vi "READDB.vi"(8 "error in (no error)":errorcluster) -> (0 "error out":errorcluster, 1 "IDS":string[](array[string]), 2 "Datos":string[][](table) caption="Result Set (from first statement with results)", 3 "Max ID":i32)   [LabVIEW 2020, in "Settings.lvlib"]
uses:
  Settings.lvlib
  <vilib>/drjdpowell/SQLite Library/SQL Connection/Open (path).vi
  <vilib>/drjdpowell/SQLite Library/SQL Connection/Open (string).vi
  <vilib>/AdvancedString/Path To Command Line String.vi
  <vilib>/drjdpowell/SQLite Library/SQL Connection/Execute SQL.vi
  <vilib>/drjdpowell/SQLite Library/SQL Connection/Connection.lvclass
  <vilib>/drjdpowell/SQLite Library/SQLite.lvlib
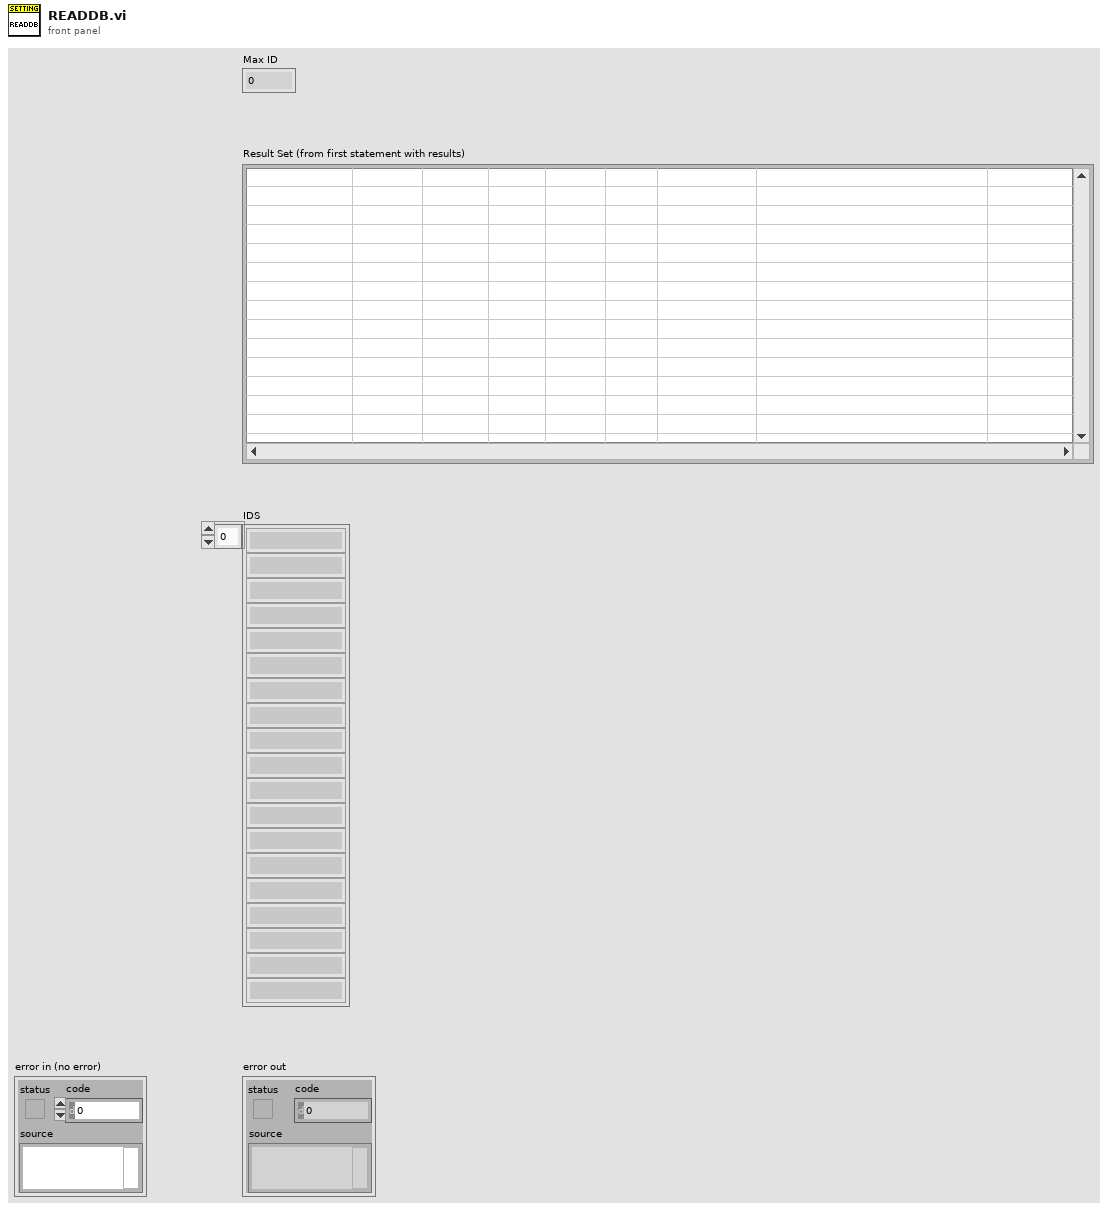
[diagram p1: front panel]
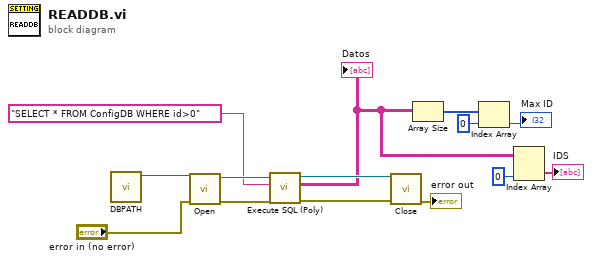
[diagram p0: block diagram]
diagram:
  n1 = call "DBPATH.vi"() -> ("appended path"=w14:path)  [unwired: 11 in]
  n2 = call-poly <vilib>:"Open.vi"("error in (no error)"="error in (no error)", "db file"=w14) -> ("error out"=w12:errorcluster, "SQLite Connection"=w11:refnum<class "Connection.lvclass">)  [unwired: 8 in]
  n3 = call-poly <vilib>:"Execute SQL (Poly).vi"("error in (no error)"=w12, "SQL"="SELECT * FROM ConfigDB WHERE id>0", "SQLite Connection in"=w11) -> ("error out"=w9:errorcluster, "Result Set"=w3:string[][], "SQLite Connection"=w10:refnum<class "Connection.lvclass">)  [unwired: 5 in, 1 out]
  "Datos" <- w3
  n4 = call-dynamic "Close.vi"("error in (no error)"=w9, "SQLite Connection in"=w10) -> ("error out"=→"error out":errorcluster)  [unwired: 9 in]
  n5 = Array Size(array=w3) -> (size(s)=w6:i32[])
  n6 = Index Array(array=w6, index=0) -> (element=→"Max ID":i32)
  n7 = Index Array(array=w3, index (col)=0 ("disabled index (col)")) -> (element=→"IDS":string[])  [unwired: 1 in]
